vi "Generate Report in PDF.vi"(8 "error in (no error)":errorcluster, 10 "Test Info":T1, 11 "Test Data":string[](array[string])) -> (0 "error out":errorcluster)   [LabVIEW 2016, in "User Interface.lvlib"]
uses:
  User Interface.lvlib
  Create Path Command.ctl
  <vilib>/addons/_office/excel.llb/Excel Easy Table (str).vi
  <vilib>/Utility/NIReport.llb/NI_report.lvclass
  <vilib>/addons/_office/NI_ReportGenerationToolkit.lvlib
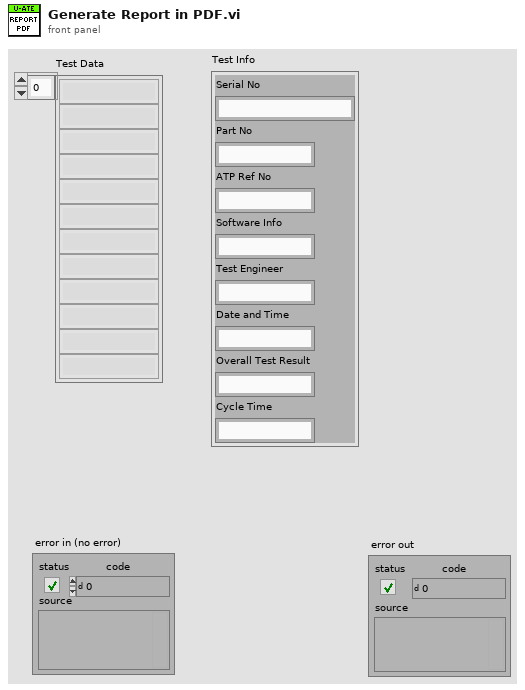
[diagram p1: front panel]
types:
  T1 = cluster{"Serial No":string, "Part No":string, "ATP Ref No":string, "Software Info":string, "Test Engineer":string, "Date and Time":string, "Overall Test Result":string, "Cycle Time":string}
  T2 = enum16{"Standard Report", "HTML", "Word", "Excel"}
  T3 = enum16{"maximized", "minimized", "normal", "no change"}
  T4 = typedef "User Interface.lvlib/Create Path Command.ctl" = enum16{"Authentication", "Hardware", "Configuration", "Calibration", "Instrument", "Test Description", "Serial Data", "ARINC Data", "CAN Data", "Data", "Report", "Action log", "Error Log"}
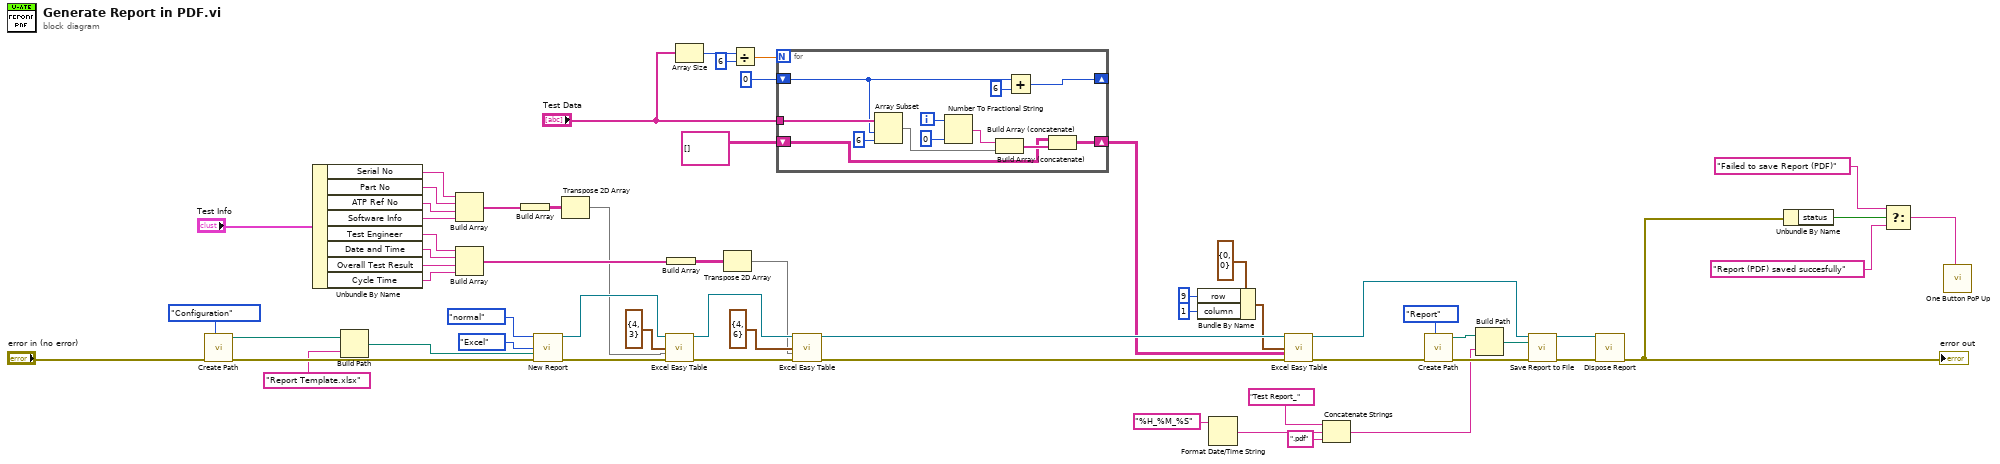
[diagram p0: block diagram]
diagram:
  n1 = call "Create Path.vi"("Path Command"=Create_Path_Command."Configuration", "error in (no error)"="error in (no error)") -> ("error out"=w55:errorcluster, "created path"=w53:path)  [unwired: 8 in]
  n2 = Unbundle By Name("Test Info") -> ("Serial No"=w26:string, "Part No"=w25:string, "ATP Ref No"=w24:string, "Software Info"=w23:string, "Test Engineer"=w22:string, "Date and Time"=w21:string, "Overall Test Result"=w20:string, "Cycle Time"=w19:string)
  n3 = Build Path(base path=w53, name or relative path="Report Template.xlsx") -> (appended path=w60:path)
  n4 = Build Array(w26, w25, w24, w23) -> (w18:string[])
  n5 = Build Array(w22, w21, w20, w19) -> (w17:string[])
  n6 = Build Array(w18) -> (w14:string[][])
  n7 = call <vilib>:"New Report.vi"("window state (normal)"=T3."normal", "report type"=T2."Excel", "template (empty)"=w60, "error in (no error)"=w55) -> ("report out"=w28:refnum<class "NI_report.lvclass">, "error out"=w32:errorcluster)  [unwired: 10 in]
  n8 = Transpose 2D Array(2D array=w14) -> (transposed array=w13:string[][])
  n9 = call-poly <vilib>:"Excel Easy Table.vi"("report in"=w28, "start (0, 0)"=cluster{"row":i32, "column":i32} {"row"=4, "column"=3}, "text data"=w13, "error in (no error)"=w32) -> ("report out"=w30:refnum<class "NI_report.lvclass">, "error out"=w29:errorcluster)  [unwired: 7 in, 3 out]
  n10 = Build Array(w17) -> (w12:string[][])
  n11 = Array Size(array="Test Data") -> (size(s)=w43:i32)
  n12 = Transpose 2D Array(2D array=w12) -> (transposed array=w11:string[][])
  n13 = Divide(x=w43, y=6) -> (x/y=w41:dbl)
  n14 = for {
    N: w41 -> [_]
    shift-right: [w63] -> w35
    shift-left: string[][] [] -> [w61]
    shift-right: [w66] -> _
    shift-left: 0 ("length") -> [w69]
    tunnel: "Test Data" -> [w72]
    i -> [w68]
    n15 = Array Subset(array=w72, index=w69, length=6) -> (w64:string[])
    n16 = Number To Fractional String(number=w68, precision (6)=i16 0) -> (F-format string=w65:string)  [unwired: 2 in]
    n17 = Build Array (concatenate)(w65, w64) -> (w62:string[])
    n18 = Add(x=w69, y=6) -> (x+y=w66:i32)
    n19 = Build Array (concatenate)(w61, w62) -> (w63:string[][])
  }
  n20 = call-poly <vilib>:"Excel Easy Table.vi"("report in"=w30, "start (0, 0)"=cluster{"row":i32, "column":i32} {"row"=4, "column"=6}, "text data"=w11, "error in (no error)"=w29) -> ("report out"=w45:refnum<class "NI_report.lvclass">, "error out"=w47:errorcluster)  [unwired: 7 in, 3 out]
  n21 = Bundle By Name(cluster=cluster{"row":i32, "column":i32} {"row"=0, "column"=0} ("start (0, 0)"), "row"=9, "column"=1) -> (w15:cluster{"row":i32, "column":i32})
  n22 = Format Date/Time String(time format string (%c)="%H_%M_%S") -> (date/time string=w3:string)  [unwired: 2 in]
  n23 = call-poly <vilib>:"Excel Easy Table.vi"("report in"=w45, "start (0, 0)"=w15, "text data"=w35, "error in (no error)"=w47) -> ("report out"=w44:refnum<class "NI_report.lvclass">, "error out"=w46:errorcluster)  [unwired: 7 in, 3 out]
  n24 = Concatenate Strings("Test Report_" ("name or relative path"), w3, ".pdf" ("string")) -> (w1:string)
  n25 = call "Create Path.vi"("Path Command"=Create_Path_Command."Report", "error in (no error)"=w46) -> ("error out"=w51:errorcluster, "created path"=w50:path)  [unwired: 8 in]
  n26 = Build Path(base path=w50, name or relative path=w1) -> (appended path=w49:path)
  n27 = call-dynamic "Save Report to File.vi"("report in"=w44, "report file path"=w49, "error in (no error)"=w51) -> ("report out"=w58:refnum<class "NI_report.lvclass">, "error out"=w59:errorcluster)  [unwired: 11 in]
  n28 = call-dynamic "Dispose Report.vi"("report in"=w58, "error in (no error)"=w59) -> ("error out"=w10:errorcluster)  [unwired: 13 in]
  "error out" <- w10
  n29 = Unbundle By Name(w10) -> ("status"=w9:bool)
  n30 = Select(t="Failed to save Report (PDF)" ("PopUpText"), s=w9, f="Report (PDF) saved succesfully" ("PopUpText")) -> (s? t:f=w6:string)
  n31 = call "One Button PoP Up.vi"("Message In"=w6) -> ()  [unwired: 11 in]
